vi "Get SDK3Handle.vi"(8 "error in (no error)":errorcluster, 11 "Handle":i32) -> (0 "error out":errorcluster, 2 "function return":u32, 3 "Handle out":i32)   [LabVIEW 2014, in "atmcd32d.lvlib"]
doc: "unsigned int WINAPI GetSDK3Handle(int * Handle);"
uses:
  atmcd32d.lvlib
  atmcd32d.dll
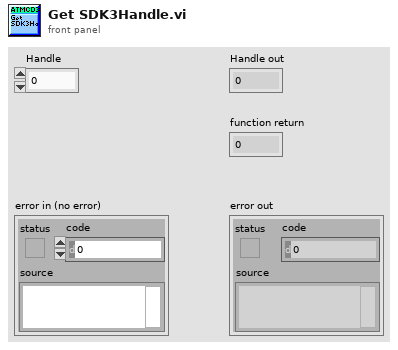
[diagram p1: front panel]
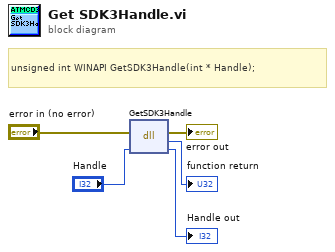
[diagram p0: block diagram]
diagram:
  # "unsigned int WINAPI GetSDK3Handle(int * Handle);"
  n1 = dll-call lib="C:/Users/Bakir/Documents/Lambda2-Testing/lib/Andorlib/atmcd32d.*" fn="GetSDK3Handle"(error in="error in (no error)", "Handle"="Handle") -> (error out=→"error out":errorcluster, →"function return":u32, "Handle"=→"Handle out":i32)  [unwired: 2 in, 1 out]
